vi "34401A DMM Close.vi"(8 "error in (no error)":errorcluster, 11 "VISA resource name":refnum<visa-resource-name>) -> (0 "error out":errorcluster)   [LabVIEW 2015]
doc: "Performs an instrument error query and terminates the software connection to the instrument."
uses:
  <instrlib>/Agilent 34401/Agilent 34401.lvlib
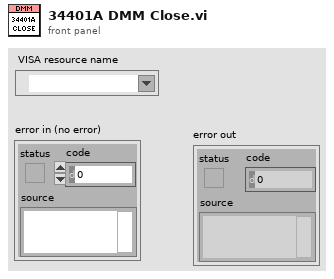
[diagram p1: front panel]
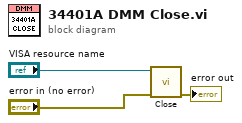
[diagram p0: block diagram]
diagram:
  n1 = call <instrlib>:"Close.vi"("error in (no error)"="error in (no error)", "VISA resource name"="VISA resource name") -> ("error out"=→"error out":errorcluster)  [unwired: 9 in]
